vi "RatioCalculation.vi"(3 "dens":sgl[][](array[numeric])) -> (0 "ratio":sgl[](array[numeric]))   [LabVIEW 2015]
uses:
  PlantType.dll
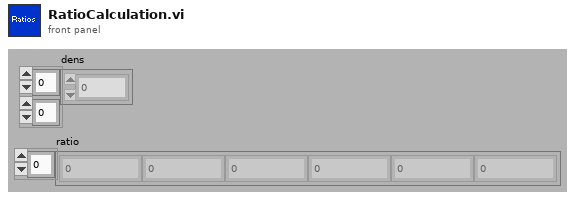
[diagram p1: front panel]
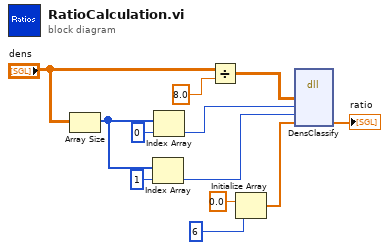
[diagram p0: block diagram]
diagram:
  n1 = Array Size(array="dens") -> (size(s)=w2:i32[])
  n2 = Index Array(array=w2, index=1) -> (element=w1:i32)
  n3 = Index Array(array=w2, index=0) -> (element=w4:i32)
  n4 = Divide(x="dens", y=sgl 8.0) -> (x/y=w7:sgl[][])
  n5 = Initialize Array(sgl 0.0 ("element"), 6 ("dimension size")) -> (w10:sgl[])
  n6 = dll-call lib="PTH2=abs E油菜汇总software\nside_features\nPlantType.dll" fn="DensClassify"("dens"=w7, "row"=w4, "col"=w1, "ratio"=w10) -> ("ratio"=→"ratio":sgl[])  [unwired: 6 in, 3 out]
